vi "fgv_stop-point_check.vi"(11 "agv curr utm":cluster{dbl, dbl}) -> (3 "stop point check":bool)   [LabVIEW 2019]
panel:
  out "distance arr":dbl[](array[numeric])
  out "stop pt update out":cluster{dbl, dbl}[](array[cluster])
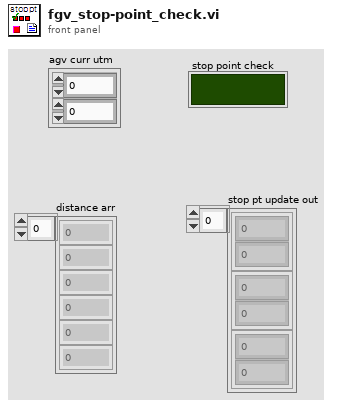
[diagram p1: front panel]
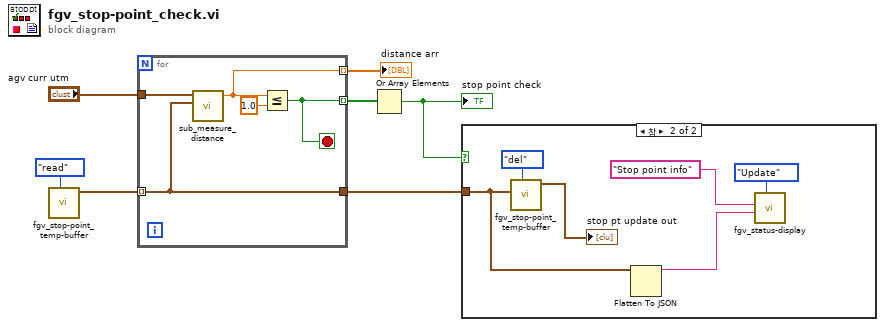
[diagram p0: block diagram]
diagram:
  n1 = call "fgv_stop-point_temp-buffer.vi"("cmd"=enum16{"init", "upload", "read", "del"}."read") -> ("stop pt update out"=w6:cluster{dbl, dbl}[])  [unwired: 10 in]
  n2 = for {
    tunnel: "agv curr utm" -> [w12]
    tunnel: w6 -> [w10] mode=indexing
    tunnel: [w9] -> w7 mode=indexing
    tunnel: [w10] -> w2
    tunnel: [w8] -> w1 mode=indexing
    stop <- w9 stop-if-true
    n3 = call "sub_measure_distance.vi"("pt 2"=w10, "pt 1"=w12) -> ("distance"=w8:dbl)  [unwired: 9 in]
    n4 = Less Or Equal?(x=w8, y=1.0) -> (x <= y?=w9:bool)
  }
  "distance arr" <- w1
  n5 = Or Array Elements(Boolean array=w7) -> (logical OR=w3:bool)
  "stop point check" <- w3
  n6 = case shown="참" w3 {
    tunnel: w2 -> [_ w15]
    frame False {
    }
    frame True {
      n7 = call "fgv_stop-point_temp-buffer.vi"("cmd"=enum16{"init", "upload", "read", "del"}."del", "arrive point"=w15) -> ("stop pt update out"=→"stop pt update out":cluster{dbl, dbl}[])  [unwired: 9 in]
      n8 = Flatten To JSON(anything=w15) -> (JSON string=w13:string)  [unwired: 2 in, 1 out]
      n9 = call "fgv_status-display.vi"("Mode"=enum16{"Initial", "Update", "Clear"}."Update", "detail"=w13, "title"="Stop point info") -> ()  [unwired: 8 in, 1 out]
    }
  }
